vi "ComputeForce.vi"(4 "Error In":errorcluster, 5 "Fixed Trap Params":T1, 6 "Steerable Trap Params":T1, 7 "Named DAQ Cluster":T3) -> (0 "Error Out":errorcluster, 1 "FxSteerTrap":dbl, 2 "FxFixedTrap":dbl, 3 "Computed Forces":T2)   [LabVIEW 2012]
panel:
  # "Compute the Forces for Both Traps"
  # "Gheorghe Chistol 09/02/13"
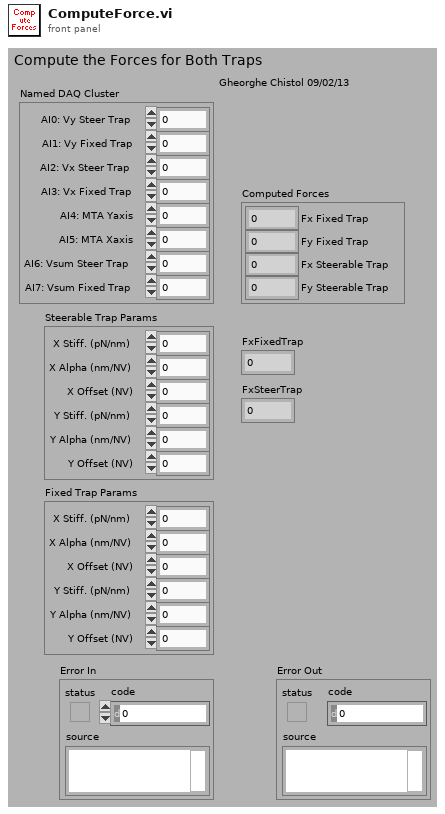
[diagram p1: front panel]
types:
  T1 = cluster{"X Stiff. (pN/nm)":dbl, "X Alpha (nm/NV)":dbl, "X Offset (NV)":dbl, "Y Stiff. (pN/nm)":dbl, "Y Alpha (nm/NV)":dbl, "Y Offset (NV)":dbl}
  T2 = cluster{"Fx Fixed Trap":dbl, "Fy Fixed Trap":dbl, "Fx Steerable Trap":dbl, "Fy Steerable Trap":dbl}
  T3 = cluster{"AI0: Vy Steer Trap":dbl, "AI1: Vy Fixed Trap":dbl, "AI2: Vx Steer Trap":dbl, "AI3: Vx Fixed Trap":dbl, "AI4: MTA Yaxis":dbl, "AI5: MTA Xaxis":dbl, "AI6: Vsum Steer Trap":dbl, "AI7: Vsum Fixed Trap":dbl}
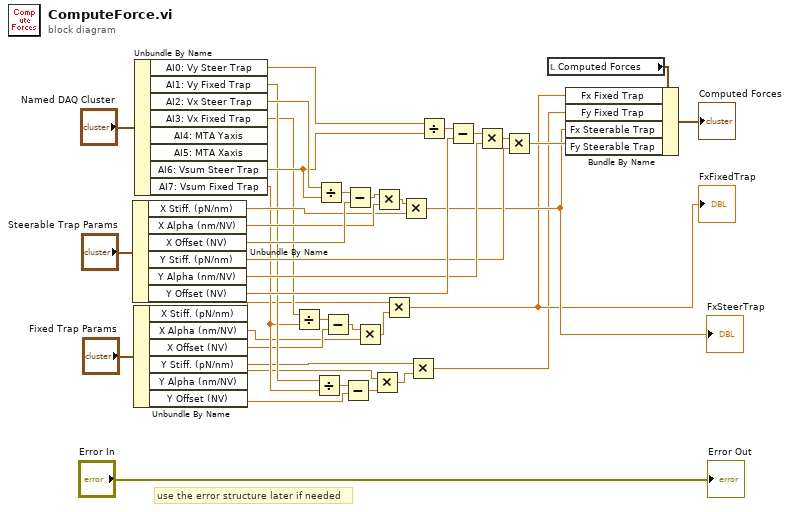
[diagram p0: block diagram]
diagram:
  # "use the error structure later if needed"
  n1 = Unbundle By Name("Steerable Trap Params") -> ("X Stiff. (pN/nm)"=w19:dbl, "X Alpha (nm/NV)"=w20:dbl, "X Offset (NV)"=w21:dbl, "Y Stiff. (pN/nm)"=w30:dbl, "Y Alpha (nm/NV)"=w31:dbl, "Y Offset (NV)"=w36:dbl)
  n2 = Unbundle By Name("Fixed Trap Params") -> ("X Stiff. (pN/nm)"=w10:dbl, "X Alpha (nm/NV)"=w8:dbl, "X Offset (NV)"=w11:dbl, "Y Stiff. (pN/nm)"=w3:dbl, "Y Alpha (nm/NV)"=w4:dbl, "Y Offset (NV)"=w6:dbl)
  n3 = Unbundle By Name("Named DAQ Cluster") -> ("AI0: Vy Steer Trap"=w35:dbl, "AI1: Vy Fixed Trap"=w14:dbl, "AI2: Vx Steer Trap"=w23:dbl, "AI3: Vx Fixed Trap"=w13:dbl, "AI6: Vsum Steer Trap"=w22:dbl, "AI7: Vsum Fixed Trap"=w12:dbl)  [unwired: 2 out]
  n4 = Divide(x=w13, y=w12) -> (x/y=w17:dbl)
  n5 = Divide(x=w14, y=w12) -> (x/y=w15:dbl)
  n6 = Divide(x=w23, y=w22) -> (x/y=w26:dbl)
  n7 = Subtract(x=w17, y=w11) -> (x-y=w16:dbl)
  n8 = Subtract(x=w15, y=w6) -> (x-y=w5:dbl)
  n9 = Subtract(x=w26, y=w21) -> (x-y=w25:dbl)
  n10 = Multiply(x=w16, y=w8) -> (x*y=w9:dbl)
  n11 = Multiply(x=w4, y=w5) -> (x*y=w2:dbl)
  n12 = Multiply(x=w25, y=w20) -> (x*y=w24:dbl)
  n13 = Multiply(x=w10, y=w9) -> (x*y=w7:dbl)
  "FxFixedTrap" <- w7
  n14 = Multiply(x=w24, y=w19) -> (x*y=w18:dbl)
  "FxSteerTrap" <- w18
  n15 = Multiply(x=w3, y=w2) -> (x*y=w1:dbl)
  n16 = Divide(x=w35, y=w22) -> (x/y=w34:dbl)
  n17 = Subtract(x=w34, y=w36) -> (x-y=w33:dbl)
  n18 = Multiply(x=w33, y=w31) -> (x*y=w32:dbl)
  n19 = Multiply(x=w32, y=w30) -> (x*y=w27:dbl)
  n20 = local read "Computed Forces"() -> (w29:T2)
  n21 = Bundle By Name(cluster=w29, "Fx Fixed Trap"=w7, "Fy Fixed Trap"=w1, "Fx Steerable Trap"=w18, "Fy Steerable Trap"=w27) -> (→"Computed Forces":T2)
  "Error Out" <- "Error In"
